vi "Configure Range Table (Spurious Emissions - Detector).vi"(0 "VISA resource name":refnum<visa-resource-name>, 5 "Detector 1 List":i32[](array[ring])=[0, 0] items=["Normal", "Average", "Peak", "Sample", "Negative Peak"], 7 "Detector 2 List":i32[](array[ring])=[0, 0] items=["Off", "Normal", "Average", "Peak", "Sample", "Negative Peak"], 11 "error in (no error)":errorcluster) -> (4 "VISA resource name out":refnum<visa-resource-name>, 15 "error out":errorcluster)   [LabVIEW 2018, in "Agilent MXA Series.lvlib"]
doc: "Configures the Detectors settings under Range Table for Spurious Emissions measurement type."
uses:
  Agilent MXA Series.lvlib
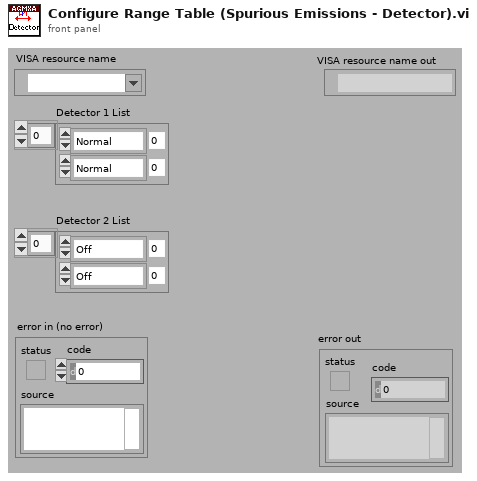
[diagram p1: front panel]
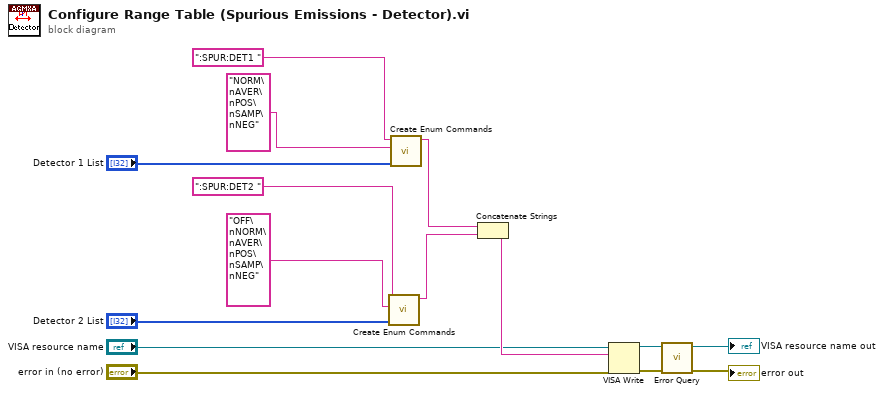
[diagram p0: block diagram]
diagram:
  n1 = call "Create Enum Commands.vi"("Enum Values"="Detector 2 List", "Multi-line Text"="OFF\nNORM\nAVER\nPOS\nSAMP\nNEG" ("multi-line string"), "Commands"=":SPUR:DET2 ") -> ("Result"=w1:string)  [unwired: 8 in]
  n2 = call "Create Enum Commands.vi"("Enum Values"="Detector 1 List", "Multi-line Text"="NORM\nAVER\nPOS\nSAMP\nNEG" ("multi-line string"), "Commands"=":SPUR:DET1 ") -> ("Result"=w2:string)  [unwired: 8 in]
  n3 = Concatenate Strings(w2, w1) -> (w15:string)
  n4 = VISA Write(VISA resource name="VISA resource name", write buffer=w15, error in (no error)="error in (no error)") -> (VISA resource name out=w11:refnum<visa-resource-name>, error out=w12:errorcluster)  [unwired: 1 out]
  n5 = call "Error Query.vi"("error in (no error)"=w12, "VISA resource name"=w11) -> ("error out"=→"error out":errorcluster, "VISA resource name out"=→"VISA resource name out":refnum<visa-resource-name>)  [unwired: 6 in, 2 out]
